vi "Create Format String.vi"(10 "Required Precision":u8=3, 11 "Base Evaluation String":string="X = %**f") -> (3 "Format String":string)   [LabVIEW 2018]
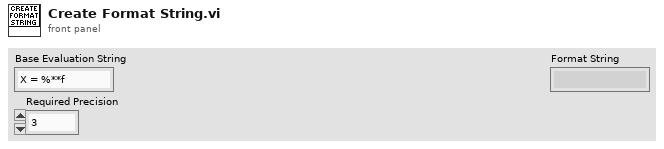
[diagram p1: front panel]
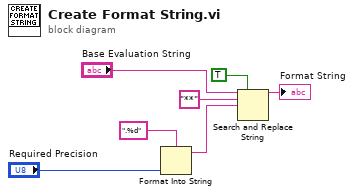
[diagram p0: block diagram]
diagram:
  n1 = Format Into String(format string=".%d", "Required Precision") -> (resulting string=w3:string)  [unwired: 2 in, 1 out]
  n2 = Search and Replace String(replace all?=TRUE ("replace all? (F)"), input string="Base Evaluation String", search string="**", replace string=w3) -> (result string=→"Format String":string)  [unwired: 4 in, 3 out]
